vi "Get Run properties.vi"(0 "Schedule in":refnum<class "Schedule.lvclass">, 5 "index":i32, 11 "error in (no error)":errorcluster) -> (2 "Run Instance":refnum<class "Run Instance.lvclass">, 3 "Repetitions":u32, 4 "Schedule out":refnum<class "Schedule.lvclass">, 6 "Script Name":string, 8 "Parameters":string[][](array[string]), 10 "Kasli Name":string, 14 "Script Path":path, 15 "error out":errorcluster)   [LabVIEW 2020, in "TALOS.lvlib" / "Run Utilities.lvlib" / "Schedule.lvclass"]
doc: "Get Script name, Script path, Script parameters, and number of cycles for the specified schedule cell"
uses:
  Schedule.lvclass
  Run Instance/Run Instance.lvclass
  Cell/Schedule Cell.lvclass
  Schedule.lvclass/Schedule.ctl
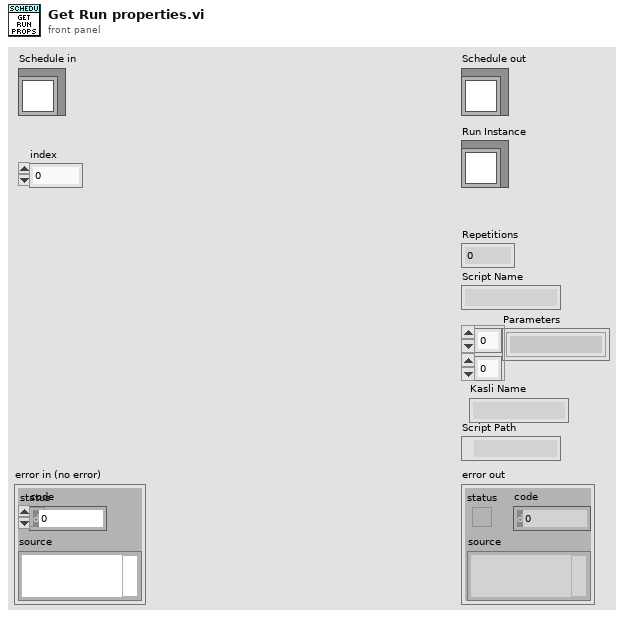
[diagram p1: front panel]
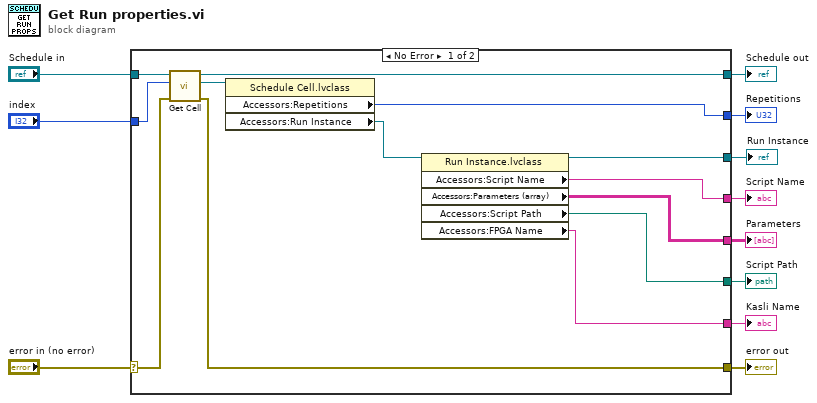
[diagram p0: block diagram]
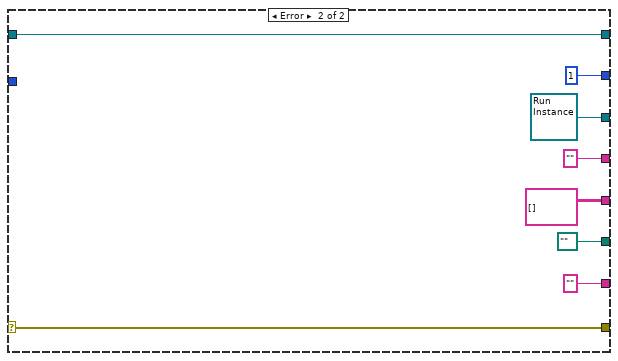
[diagram p2: hidden frame]
diagram:
  n1 = case shown="No Error" "error in (no error)" {
    selector: "error in (no error)" -> [w21 w32]
    tunnel: [w20 w32] -> w10
    tunnel: [w23 w31] -> w8
    tunnel: "Schedule in" -> [w24 w31]
    tunnel: "index" -> [w22 _]
    tunnel: [w13 u32 1 ("Repetitions")] -> w6
    tunnel: [w19 "" ("Accessors:Script Name")] -> w5
    tunnel: [w18 string[][] [] ("Accessors:Parameters")] -> w4
    tunnel: [w17 path "" ("Accessors:Script Path")] -> w3
    tunnel: [w16 "" ("Accessors:Kasli Name")] -> w2
    tunnel: [w12 refnum<class "Run Instance.lvclass"> refnum ("Run Instance")] -> w1
    frame No Error {
      n2 = call-dynamic "Get Cell.vi"("error in (no error)"=w21, "index"=w22, "Schedule in"=w24) -> ("error out"=w20:errorcluster, "Schedule Cell"=w15:refnum<class "Schedule Cell.lvclass">, "Schedule out"=w23:refnum<class "Schedule.lvclass">)  [unwired: 6 in]
      n3 = property class="Schedule Cell.lvclass"(reference=w15) -> ("Accessors:Repetitions"=w13:u32, "Accessors:Run Instance"=w14:refnum<class "Run Instance.lvclass">)  [unwired: 1 in, 2 out]
      n4 = property class="Run Instance.lvclass"(reference=w14) -> (reference out=w12:refnum<class "Run Instance.lvclass">, "Accessors:Script Name"=w19:string, "Accessors:Parameters (array)"=w18:string[][], "Accessors:Script Path"=w17:path, "Accessors:FPGA Name"=w16:string)  [unwired: 1 in, 1 out]
    }
    frame Error {
    }
  }
  "error out" <- w10
  "Schedule out" <- w8
  "Repetitions" <- w6
  "Script Name" <- w5
  "Parameters" <- w4
  "Script Path" <- w3
  "Kasli Name" <- w2
  "Run Instance" <- w1
